vi "ATS_BoardsInSystem.vi"(7 "sid_In":u32) -> (2 "Num_Of_Boards":u32, 3 "sid_Out":u32)   [LabVIEW 2010]
doc: "_____AlazarTech, Scope_____\n\nReturn the total number of configured devices for a given system.\n\nInput:\n\"sid_In\" = system identification number. Must be >0 \n\nOutput:\n\"sid_Out\" = system identification read\n\"Num_Board\" = number of boards in system (configured devices)"
uses:
  ATSApi.dll
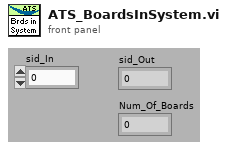
[diagram p1: front panel]
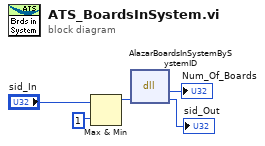
[diagram p0: block diagram]
diagram:
  n1 = Max & Min(x="sid_In", y=u32 1) -> (max(x,y)=w2:u32)  [unwired: 1 out]
  n2 = dll-call lib="ATSApi.dll" fn="AlazarBoardsInSystemBySystemID"("sid"=w2) -> (→"Num_Of_Boards":u32, "sid"=→"sid_Out":u32)  [unwired: 3 in, 2 out]
